vi "Playground.vi"() -> ()   [LabVIEW 2016]
uses:
  Source/Engine/Classes/Interface/DSF.Engine.Interface.Builder.Command Data.ctl
  Source/Engine/Classes/Interface/DSF.Engine.Interface.Builder.Command.ctl
  Source/Engine/Classes/Cache/DSF.Engine.Memory.Cache.Framework.lvclass
  Source/Engine/Classes/Thread Parameters/Thread Parameters.lvclass/Thread Parameters.ctl
  Source/Engine/Classes/Interface/DSF.Engine.Interface.Builder.Write.Command.vi
  Source/Engine/Classes/Thread Parameters/Thread Parameters.lvclass
  Source/Engine/Classes/Builder/DSF.Engine.Builder.lvclass
  Source/Engine/Classes/Interface/DSF.Engine.Interface.Builder.lvclass
panel:
  out "error out":errorcluster
  in  "command":T1
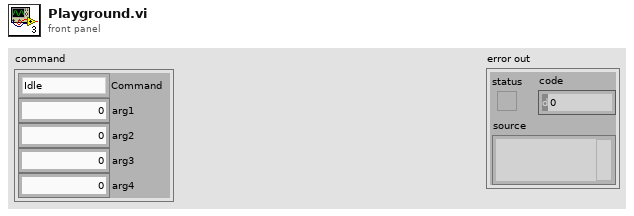
[diagram p1: front panel]
types:
  T1 = typedef "DSF.Engine.lvlib/DSF.Engine.Interface.Builder.lvclass/DSF.Engine.Interface.Builder.Command Data.ctl" = cluster{"Command":T2, "arg1":i32, "arg2":i32, "arg3":i32, "arg4":i32}
  T2 = typedef "DSF.Engine.lvlib/DSF.Engine.Interface.Builder.lvclass/DSF.Engine.Interface.Builder.Command.ctl" = enum8{"Idle", "Initialize", "Build Buffer", "Parse Buffer", "Shutdown"}
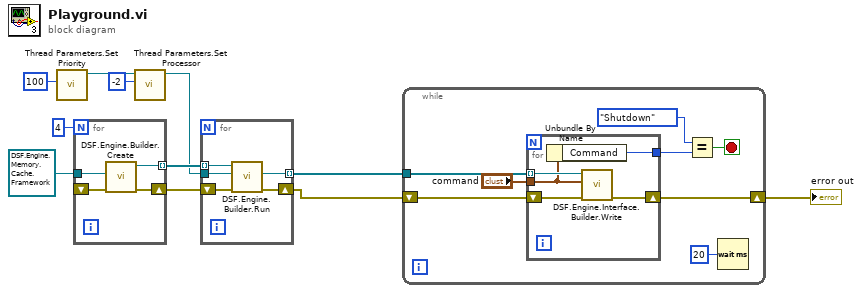
[diagram p0: block diagram]
diagram:
  n1 = call "Thread Parameters.Set Priority.vi"("Priority"=100) -> ("Thread Parameters out"=w10:refnum<class "Thread Parameters.lvclass">)  [unwired: 10 in]
  n2 = for {
    N: 4 -> [_]
    tunnel: refnum<class "DSF.Engine.Memory.Cache.Framework.lvclass"> refnum ("Framework Cache") -> [w15]
    tunnel: [w14] -> w5 mode=indexing
    shift-right: [w13] -> w4
    shift-left: _ -> [w12]
    n3 = call "DSF.Engine.Builder.Create.vi"("error in (no error)"=w12, "Framework Cache"=w15) -> ("error out"=w13:errorcluster, "Builder"=w14:refnum<class "DSF.Engine.Builder.lvclass">)  [unwired: 8 in]
  }
  n4 = call "Thread Parameters.Set Processor.vi"("Processor"=-2, "Thread Parameters in"=w10) -> ("Thread Parameters out"=w1:refnum<class "Thread Parameters.lvclass">)  [unwired: 9 in]
  n5 = for {
    shift-right: [w19] -> w3
    shift-left: w4 -> [w20]
    tunnel: w5 -> [w18] mode=indexing
    tunnel: [w17] -> w2 mode=indexing
    tunnel: w1 -> [w16]
    n6 = call "DSF.Engine.Builder.Run.vi"("error in (no error)"=w20, "Thread Parameters"=w16, "Builder in"=w18) -> ("error out"=w19:errorcluster, "Builder Interface"=w17:refnum<class "DSF.Engine.Interface.Builder.lvclass">)  [unwired: 6 in, 1 out]
  }
  n7 = while {
    tunnel: w2 -> [w28]
    shift-right: [w24] -> w7
    shift-left: w3 -> [w27]
    stop <- w21 stop-if-true
    n8 = for {
      tunnel: w28 -> [w33] mode=indexing
      tunnel: "command" -> [w30]
      shift-right: [w31] -> w24
      shift-left: w27 -> [w32]
      tunnel: [w29] -> w23
      n9 = Unbundle By Name(w30) -> ("Command"=w29:T2)
      n10 = call-poly "DSF.Engine.Interface.Builder.Write.vi"("error in (no error)"=w32, "command"=w30, "Builder Interface in"=w33) -> ("error out"=w31:errorcluster)  [unwired: 6 in, 2 out]
    }
    n11 = Equal?(x=DSF.Engine.Interface.Builder.Command."Shutdown", y=w23) -> (x = y?=w21:bool)
    n12 = Wait (ms)(milliseconds to wait=u32 20) -> ()  [unwired: 1 out]
  }
  "error out" <- w7
